vi "transmitter.vi"() -> ()   [LabVIEW 2013]
uses:
  <instrlib>/niUSRP/niUSRP Write Tx Data (CDB).vi
panel:
  in  "active antenna":string
  in  "gain":dbl format="%#_6f"
  in  "carrier frequency":dbl=100000.0 format="%#_6p"
  in  "IQ rate":dbl=100000.0 format="%#_6p"
  in  "waveform size":i32
  in  "device names":refnum<k15>
  in  "stop":bool
  out "coerced gain":dbl format="%#_6f"
  out "coerced carrier frequency":dbl=100000.0 format="%#_6p"
  out "coerced IQ rate":dbl=100000.0 format="%#_6p"
  out "error out":errorcluster
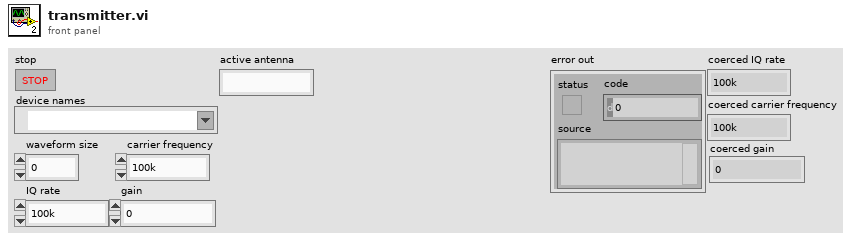
[diagram p1: front panel]
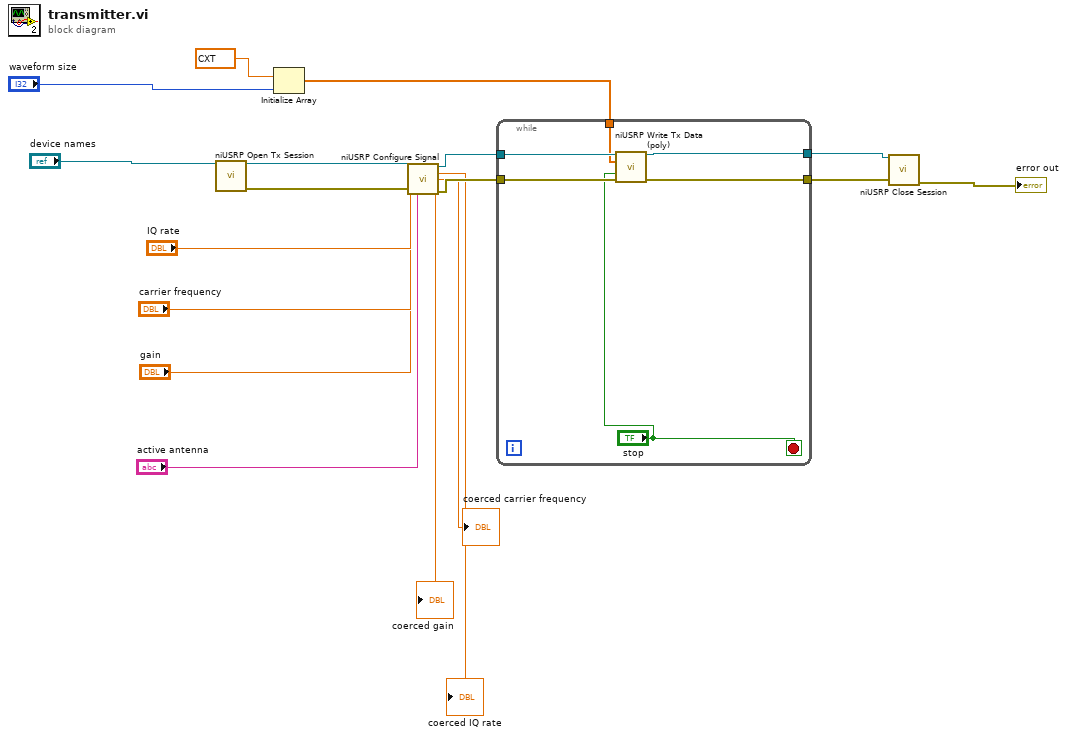
[diagram p0: block diagram]
diagram:
  n1 = call <instrlib>:"niUSRP Open Tx Session.vi"("device names"="device names") -> ("session handle out"=w17:refnum<k15>, "error out"=w14:errorcluster)  [unwired: 13 in]
  n2 = Initialize Array "Initialize Array"(cxt 1.0+0.0i ("element"), "waveform size") -> (w8:cxt[])
  n3 = call <instrlib>:"niUSRP Configure Signal.vi"("session handle"=w17, "IQ rate"="IQ rate", "carrier frequency"="carrier frequency", "gain"="gain", "error in (no error)"=w14, "active antenna"="active antenna") -> ("session handle out"=w16:refnum<k15>, "coerced IQ rate"=→"coerced IQ rate":dbl, "coerced carrier frequency"=→"coerced carrier frequency":dbl, "coerced gain"=→"coerced gain":dbl, "error out"=w13:errorcluster)  [unwired: 5 in]
  n4 = while {
    tunnel: w16 -> [w24]
    tunnel: [w23] -> w15
    tunnel: w13 -> [w22]
    tunnel: [w21] -> w12
    tunnel: w8 -> [w19]
    stop <- "stop" stop-if-true
    n5 = call-poly <instrlib>:"niUSRP Write Tx Data (poly).vi"("session handle"=w24, "data"=w19, "end of data?"="stop", "error in (no error)"=w22) -> ("session handle out"=w23:refnum<k15>, "error out"=w21:errorcluster)  [unwired: 10 in]
  }
  n6 = call <instrlib>:"niUSRP Close Session.vi"("session handle"=w15, "error in (no error)"=w12) -> ("error out"=→"error out":errorcluster)  [unwired: 13 in]
